vi "Acquire_wp_nodt.vi"(0 "Ch Armed Reg":refnum<k21>="Register 1", 1 "Command FIFO":refnum<k21>, 3 "Circular Buffer Mem":refnum<k21>, 4 "circular buffer length":u32=300, 5 "FPGA I/O In":refnum<k21>="IO Module\\AI A0", 7 "channel on/off":bool, 9 "Trigger":i16=1500, 10 "Timing FIFO":refnum<k21>, 11 "Samples to Acquire":u32=100, 13 "Is Test Pulse?":bool, 14 "# of pretrigger":u32=15, 15 "timing":u64) -> ()   [LabVIEW 2012]
uses:
  <vilib>/rvi/DataTransferAndStorage/Container/Common/niFpgaContainerExecOnDevCompGetState.vi
  <vilib>/rvi/Memory/Memory_Emulation/nirvimemoryEmulationManagerCache_GetValue.vi
  <vilib>/rvi/Memory/Memory_Emulation/niFpgaMemoryEmulationValidateCache.vi
  <vilib>/rvi/DataTransferAndStorage/Container/Common/niFpgaContainerGetUniqueNameForEmu.vi
  <vilib>/rvi/Memory/Memory_Emulation/nirvimemoryEmulationManagerCache_InsertValue.vi
  <vilib>/rvi/eio/common/nirviEmuTemplateMethod_errors.vi
  <vilib>/rvi/Emulation/niFpgaSctlEmulationGetInTimedLoop.vi
  <vilib>/rvi/FIFO/Fifo_Resource/nirvififoEmulationSetSize.vi
  <vilib>/rvi/errors/niFpgaSetErrorForExecOnDevCompSimple.vi
  <vilib>/rvi/eio/common/nirviEmuReportErrorAndStop.vi
  <vilib>/rvi/Emulation/niFpgaSctlEmulationFifoFullMgr.vi
  <vilib>/rvi/Emulation/niFpgaSctlEmulationResourceMgr.vi
  <vilib>/rvi/interface/RandomDataEmulation/nirviRandomDataFPGAFIFO.vi
  <vilib>/rvi/interface/RandomDataEmulation/niFpgaRandomDataHandleErrors.vi
  <vilib>/rvi/DataTransferAndStorage/Container/XNode/niFpgaContainer.xnode
  <vilib>/rvi/DataTransferAndStorage/Register/Emulation/niFpgaRegisterEmulationRefIn.vi
  <vilib>/eio/EIONode/EIONode.xnode
  <vilib>/rvi/FIFO/Fifo_Resource/niFpgaFifoEmulationRefIn.vi
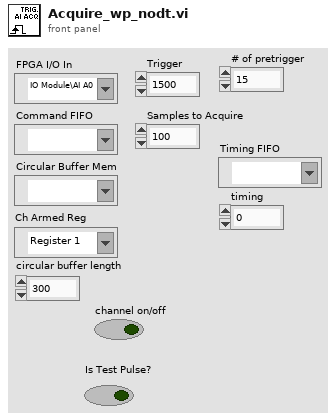
[diagram p1: front panel]
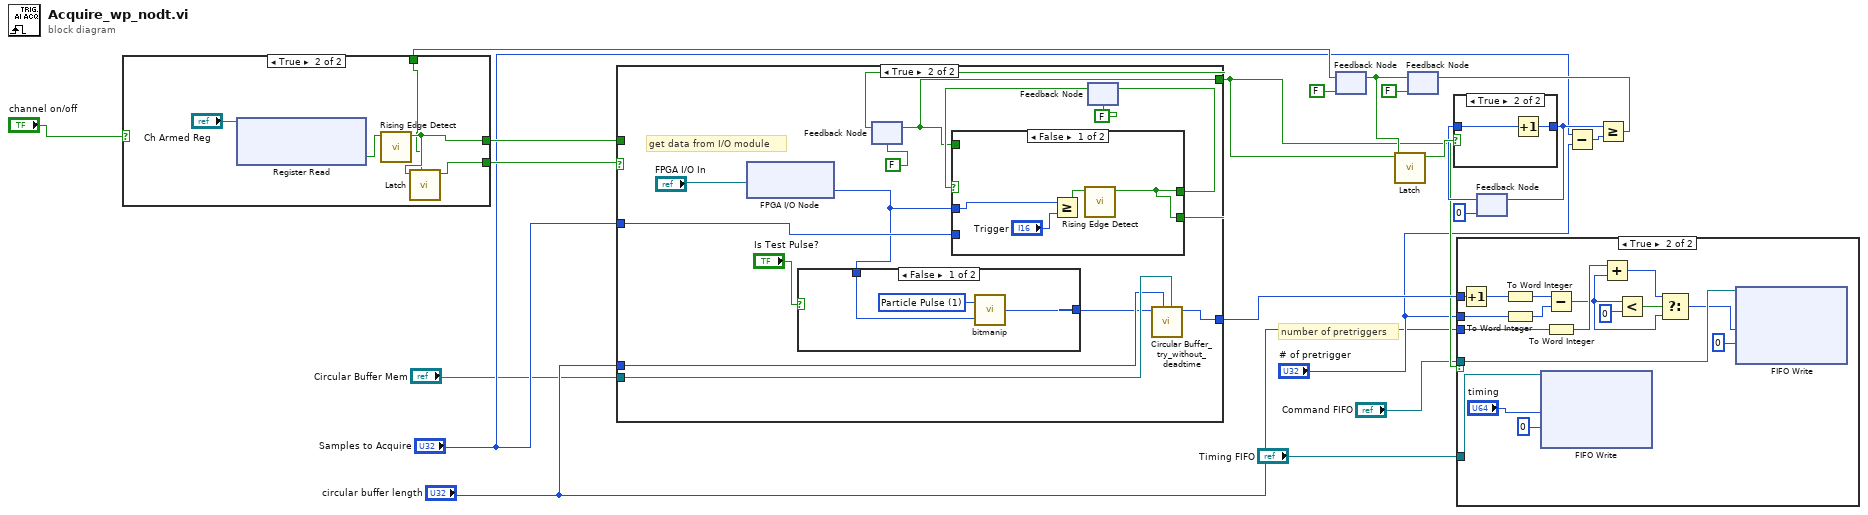
[diagram p0: block diagram]
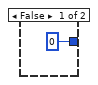
[diagram p3: hidden frame]
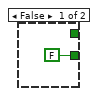
[diagram p4: hidden frame]
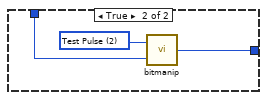
[diagram p6: hidden frame]
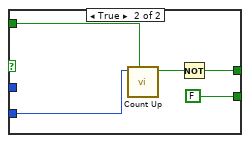
[diagram p7: hidden frame]
diagram:
  # "number of pretriggers"
  n1 = feedback #1(FALSE) -> (w16:bool)
  n2 = case shown="True" "channel on/off" {
    tunnel: [FALSE ("Output") w26] -> w21
    tunnel: [_ w27] -> w20
    tunnel: w16 -> [_ w25]
    frame False {
    }
    frame True {
      n3 = xnode ("Register Read")("Register In"="Ch Armed Reg") -> ("Data"=w23:bool)  [unwired: 1 out]
      n4 = call "Rising Edge Detect.vi"("Input"=w23) -> ("Rising Edge"=w27:bool)  [unwired: 10 in]
      n5 = call "Latch.vi"("Reset"=w25, "Input"=w27) -> ("Output"=w26:bool)  [unwired: 9 in]
    }
  }
  n6 = case shown="True" w21 {
    tunnel: "Circular Buffer Mem" -> [_ w41]
    tunnel: "circular buffer length" -> [_ w37]
    tunnel: [_ w40] -> w19
    tunnel: w20 -> [_ _]
    tunnel: "Samples to Acquire" -> [_ w36]
    tunnel: [_ w32] -> w8
    frame False {
    }
    frame True {
      # "get data from I/O module"
      n7 = xnode "FPGA I/O Node"("FPGA I/O In"="FPGA I/O In") -> ("I/O Item"=w28:i16)  [unwired: 1 out]
      n8 = case shown="False" "Is Test Pulse?" {
        tunnel: w28 -> [w43 w46]
        tunnel: [w42 w45] -> w30
        frame False {
          w44 = u16 1 items=["Header Information", "Particle Pulse", "Test Pulse"] ("Pulse Type")
          n9 = call "bitmanip.vi"("Pulse Type"=w44, "Integer to be written"=w43) -> ("Integer Written"=w42:i16)  [unwired: 2 in]
        }
        frame True {
          w47 = u16 2 items=["Header Information", "Particle Pulse", "Test Pulse"] ("Pulse Type")
          n10 = call "bitmanip.vi"("Pulse Type"=w47, "Integer to be written"=w46) -> ("Integer Written"=w45:i16)  [unwired: 2 in]
        }
      }
      n11 = feedback #2(FALSE) -> (w32:bool)
      n12 = feedback #3(FALSE) -> (w35:bool)
      n13 = case shown="False" w35 {
        tunnel: w28 -> [w51 _]
        tunnel: w36 -> [_ w56]
        tunnel: w32 -> [_ w55]
        tunnel: [w49 w53] -> w34
        tunnel: [w49 FALSE] -> w33
        frame False {
          n14 = Greater Or Equal?(x=w51, y="Trigger") -> (x >= y?=w50:bool)
          n15 = call "Rising Edge Detect.vi"("Input"=w50) -> ("Rising Edge"=w49:bool)  [unwired: 10 in]
        }
        frame True {
          n16 = call "Count Up.vi"("Reset?"=w55, "goal"=w56) -> ("Count Met"=w54:bool)  [unwired: 8 in, 1 out]
          n17 = Not(x=w54) -> (.not. x?=w53:bool)
        }
      }
      n18 = feedback-in #2(w33) -> ()
      n19 = feedback-in #3(w34) -> ()
      n20 = call "Circular Buffer_try_without_deadtime.vi"("Refnum in"=w41, "circular buffer length"=w37, "Data"=w30) -> ("Address"=w40:u16)  [unwired: 8 in]
    }
  }
  n21 = feedback #4(FALSE) -> (w14:bool)
  n22 = feedback-in #1(w14) -> ()
  n23 = call "Latch.vi"("Reset"=w14, "Input"=w8) -> ("Output"=w12:bool)  [unwired: 9 in]
  n24 = case shown="True" w8 {
    tunnel: "Command FIFO" -> [_ w73]
    tunnel: "Timing FIFO" -> [_ w72]
    tunnel: w19 -> [_ w61]
    tunnel: "circular buffer length" -> [_ w59]
    tunnel: "# of pretrigger" -> [_ w58]
    frame False {
    }
    frame True {
      n25 = Increment(x=w61) -> (x+1=w67:u16)
      n26 = To Word Integer(number=w67) -> (16bit integer=w68:i16)
      n27 = To Word Integer(number=w58) -> (16bit integer=w69:i16)
      n28 = xnode ("FIFO Write")("Element"="timing", "Timeout"=0, "FIFO In"=w72) -> ()  [unwired: 2 out]
      n29 = Subtract(x=w68, y=w69) -> (x-y=w65:i16)
      n30 = To Word Integer(number=w59) -> (16bit integer=w66:i16)
      n31 = Add(x=w66, y=w65) -> (x+y=w64:i16)
      n32 = Less?(x=w65, y=i16 0) -> (x < y?=w62:bool)
      n33 = Select(t=w64, s=w62, f=w65) -> (s? t:f=w60:i16)
      n34 = xnode ("FIFO Write")("Element"=w60, "Timeout"=0, "FIFO In"=w73) -> ()  [unwired: 2 out]
    }
  }
  n35 = feedback #5(u32 0) -> (w11:u32)
  n36 = case shown="True" w12 {
    tunnel: w11 -> [_ w76]
    tunnel: [i16 0 w75] -> w9
    frame False {
    }
    frame True {
      n37 = Increment(x=w76) -> (x+1=w75:u32)
    }
  }
  n38 = feedback-in #5(w9) -> ()
  n39 = Subtract(x="Samples to Acquire", y="# of pretrigger") -> (x-y=w10:u32)
  n40 = Greater Or Equal?(x=w9, y=w10) -> (x >= y?=w15:bool)
  n41 = feedback-in #4(w15) -> ()
